vi "PSDS_Create Object.vi"(8 "error in (no error)":errorcluster, 11 "Object Name":string) -> (0 "error out":errorcluster, 3 "Object Name Out":string)   [LabVIEW 2016]
panel:
  # "Data Out"
  # "Data In"
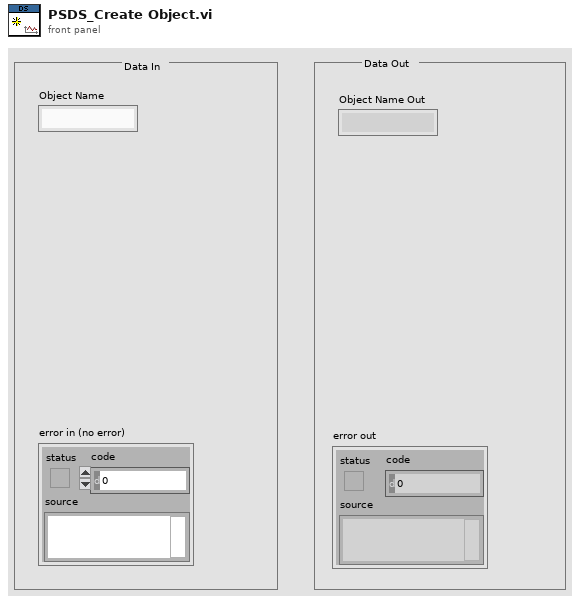
[diagram p1: front panel]
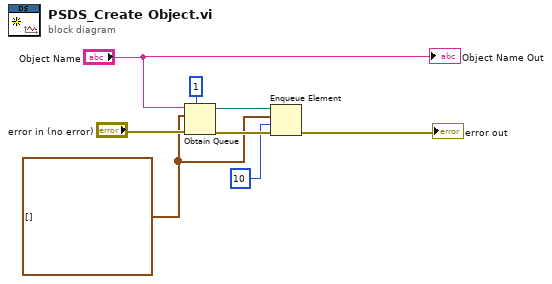
[diagram p0: block diagram]
diagram:
  w2 = waveform(dbl)[] [] ("Wave")
  n1 = Obtain Queue(max queue size (-1, unlimited)=1 ("队列最大值（-1，无限）"), name (unnamed)="Object Name", element data type=w2, error in (no error)="error in (no error)") -> (queue out=w7:refnum<queue>, error out=w6:errorcluster)  [unwired: 1 in, 1 out]
  n2 = Enqueue Element(queue=w7, element=w2, timeout in ms (-1)=10 ("超时毫秒(-1)"), error in (no error)=w6) -> (error out=→"error out":errorcluster)  [unwired: 2 out]
  "Object Name Out" <- "Object Name"
